vi "GetText.vi"(8 "error in":errorcluster, 11 "node in":refnum<class "CustomDevice.lvclass">) -> (0 "error out":errorcluster, 1 "additional text":string, 2 "text":string, 3 "node out":refnum<class "CustomDevice.lvclass">, 4 "glyph":string)   [LabVIEW 2015, in "CustomDevice.lvclass"]
doc: "Returns the text representation of the node used for the tree control."
uses:
  CustomDevice.lvclass
  CustomDevice.lvclass/CustomDevice.ctl
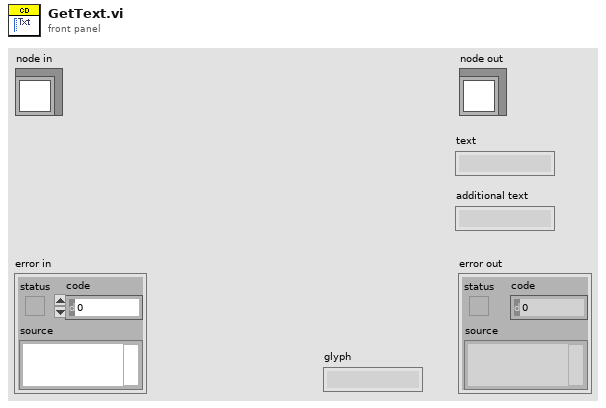
[diagram p1: front panel]
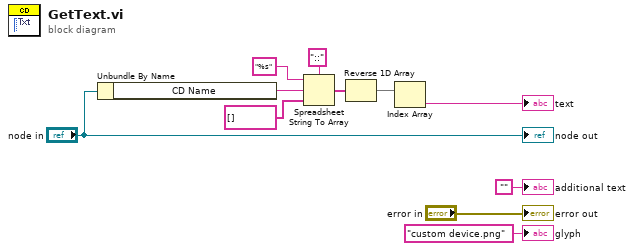
[diagram p0: block diagram]
diagram:
  n1 = Unbundle By Name("node in") -> ("CD Name"=w7:string)
  n2 = Spreadsheet String To Array(delimiter (Tab)="::", format string="%s", spreadsheet string=w7, array type (2D Dbl)=string[] []) -> (array=w4:string[])
  n3 = Reverse 1D Array(array=w4) -> (reversed array=w3:string[])
  n4 = Index Array(array=w3) -> (element=→"text":string)  [unwired: 1 in]
  "error out" <- "error in"
  "node out" <- "node in"
  "additional text" <- ""
  "glyph" <- "custom device.png" ("glyph")
